vi "Lidar Processing.vi"(7 "robotPosition":T2, 8 "Direction 2":dbl[](array[numeric]), 9 "Magnitude 2":dbl[](array[numeric]), 10 "Direction":dbl[](array[numeric]), 11 "Magnitude":dbl[](array[numeric])) -> (0 "closeLidar":cluster{dbl, dbl}[](array[cluster]), 3 "Lidar Data":cluster{dbl[], dbl[]}[](graph), 4 "plotPoints":cluster{dbl, dbl}[](array[cluster]), 5 "Error":T1)   [LabVIEW 2015]
panel:
  out "Local Lidar":cluster{dbl[], dbl[]}(graph)
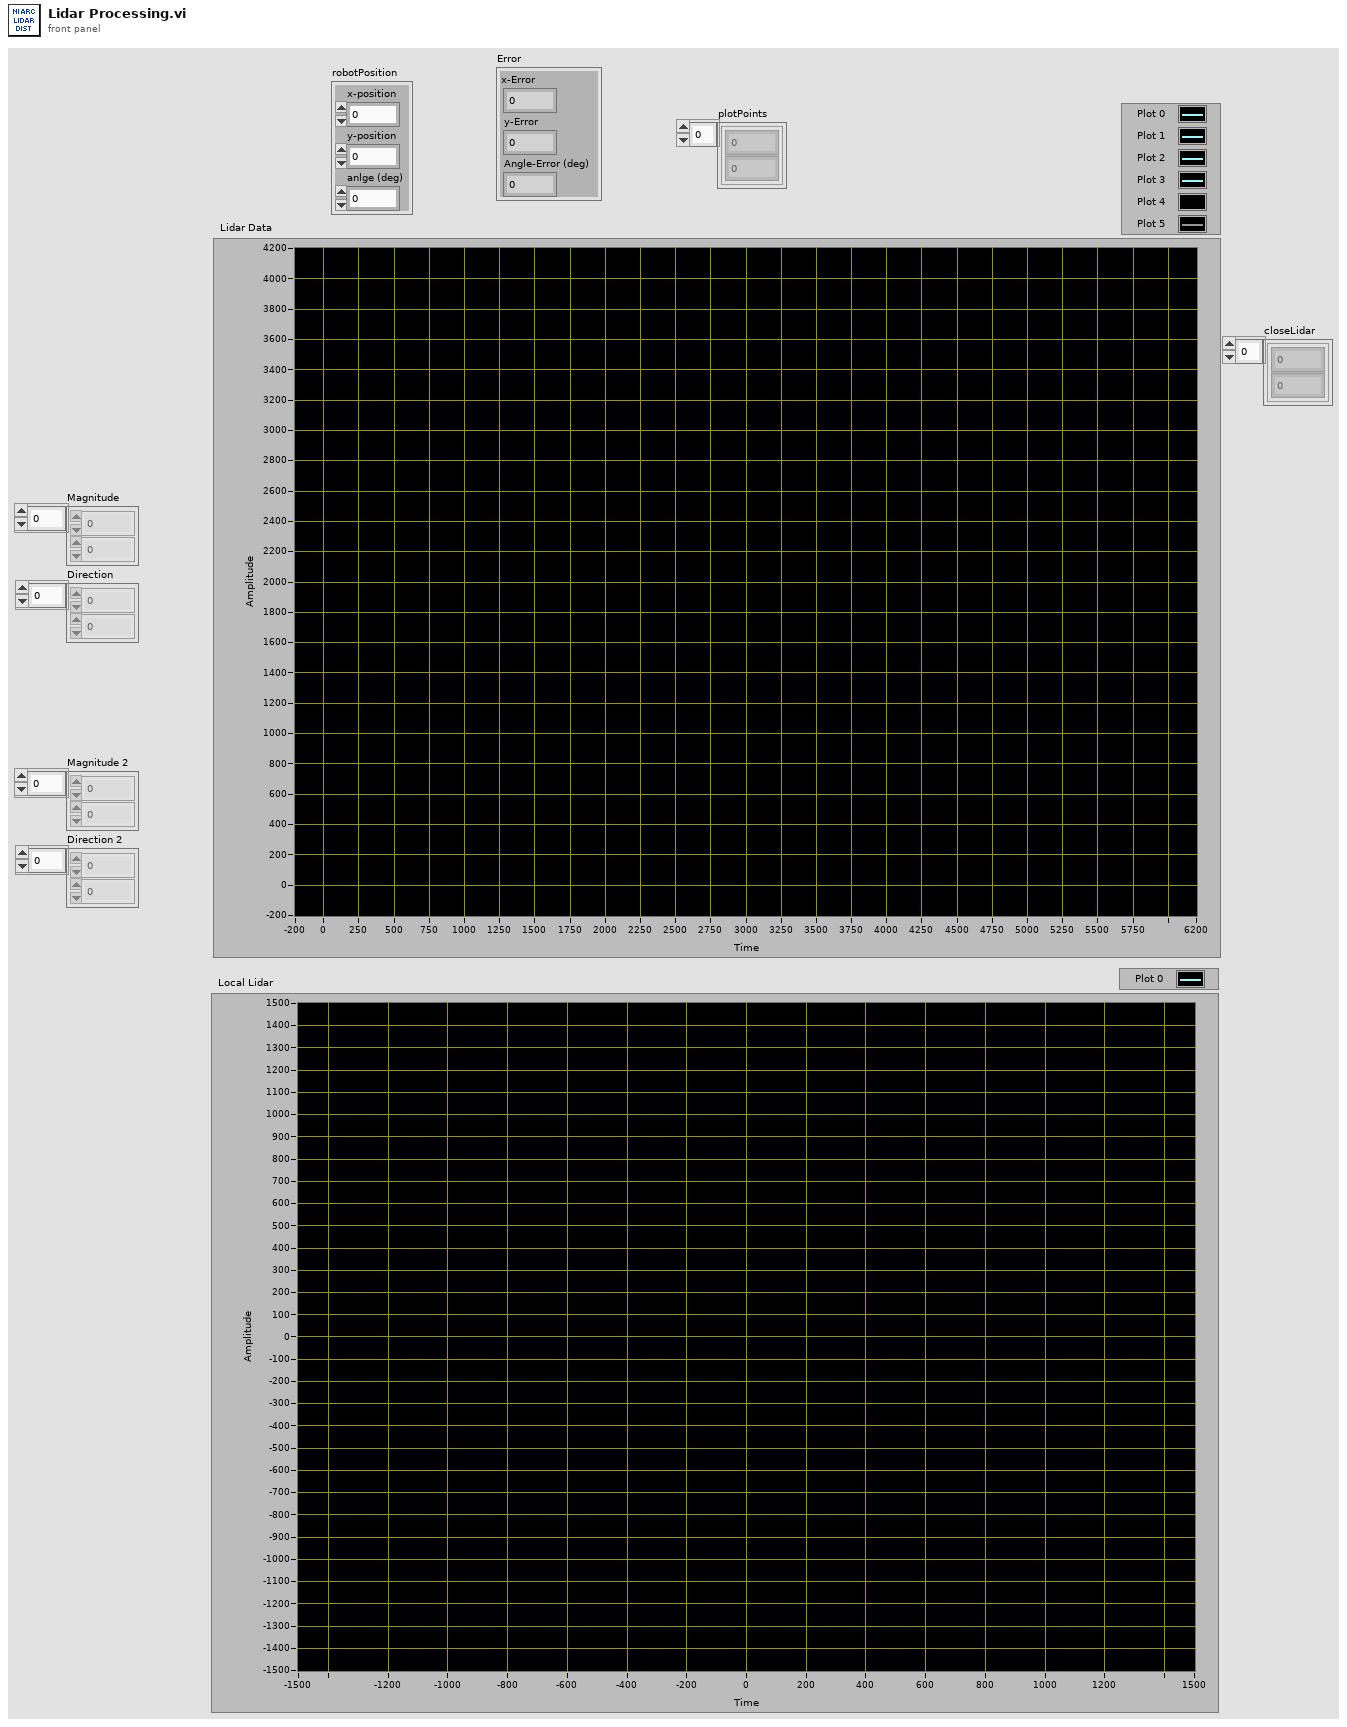
[diagram p1: front panel]
types:
  T1 = cluster{"x-Error":dbl, "y-Error":dbl, "Angle-Error (deg)":dbl}
  T2 = cluster{"x-position":dbl, "y-position":dbl, "anlge (deg)":dbl}
  T3 = cluster{"Line Segment":cluster{"Point 1":cluster{"X":sgl, "Y":sgl}, "Point 2":cluster{"X":sgl, "Y":sgl}}, "Residual":dbl, "Valid Fit?":bool}[]
  T4 = cluster{"t":dbl, "t":dbl, "detectedAngle (deg)":dbl}
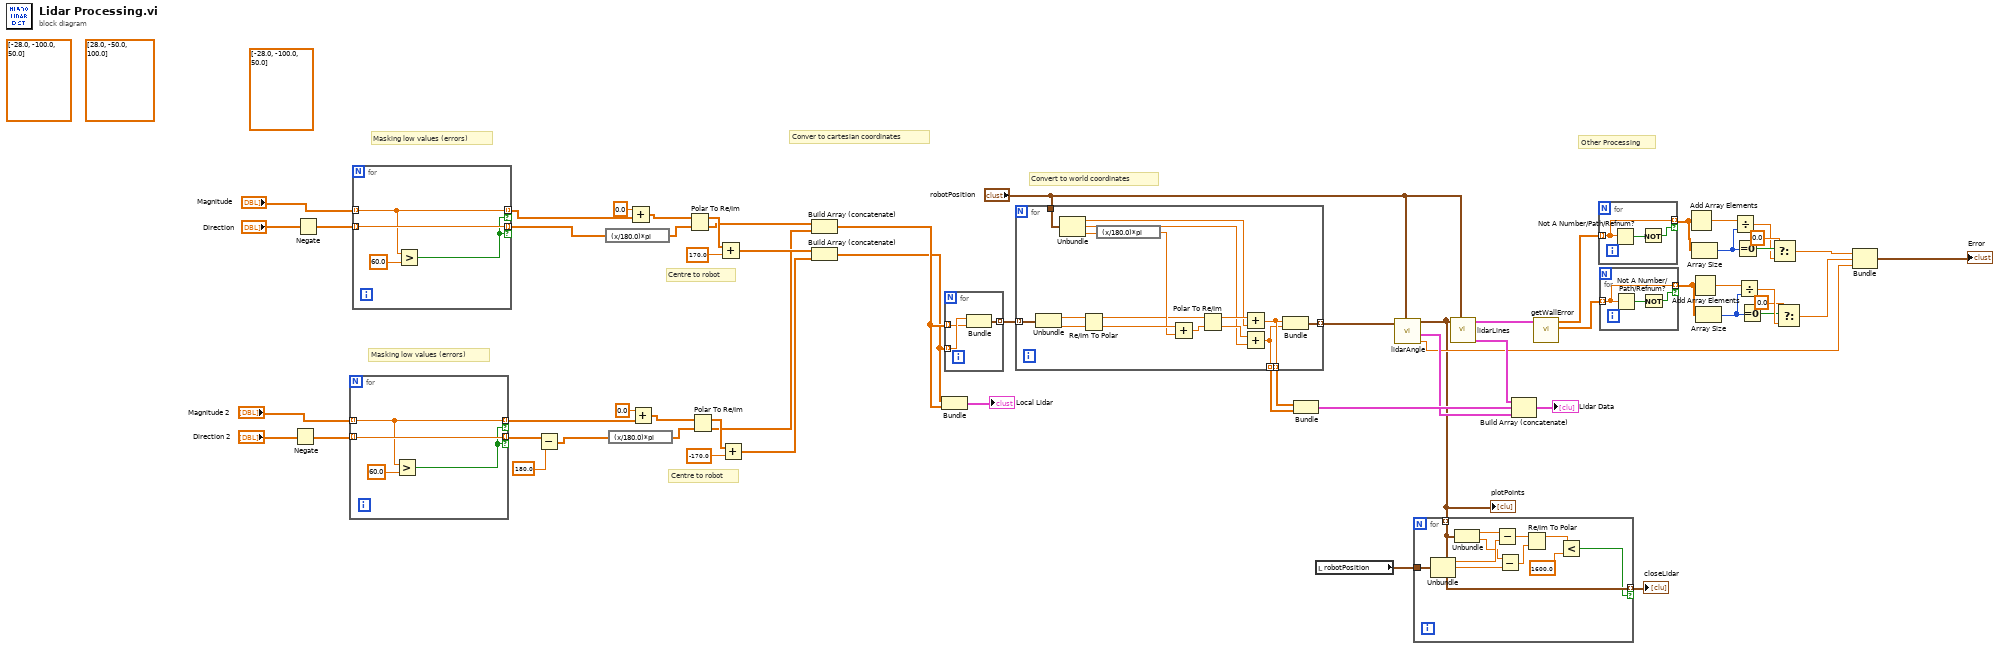
[diagram p0: block diagram]
diagram:
  (unwired) sgl[] [-28.0, -100.0, 50.0] ("Array")
  (unwired) sgl[] [28.0, -50.0, 100.0] ("Array 2")
  (unwired) sgl[] [-28.0, -100.0, 50.0] ("Array")
  # "Centre to robot"
  # "Masking low values (errors)"
  # "Convert to world coordinates"
  # "Other Processing"
  # "Masking low values (errors)"
  # "Conver to cartesian coordinates"
  # "Centre to robot"
  n1 = Negate(x="Direction 2") -> (-x=w21:dbl[])
  n2 = Negate(x="Direction") -> (-x=w56:dbl[])
  n3 = for {
    tunnel: "Magnitude 2" -> [w62] mode=indexing
    tunnel: w21 -> [w64] mode=indexing
    tunnel: [w62] -> w13 mode=indexing if=w61
    tunnel: [w64] -> w12 mode=indexing if=w61
    n4 = Greater?(x=w62, y=60.0) -> (0:w61:bool)
  }
  n5 = for {
    tunnel: "Magnitude" -> [w66] mode=indexing
    tunnel: w56 -> [w68] mode=indexing
    tunnel: [w66] -> w55 mode=indexing if=w65
    tunnel: [w68] -> w54 mode=indexing if=w65
    n6 = Greater?(x=w66, y=60.0) -> (0:w65:bool)
  }
  n7 = Subtract(x=w12, y=180.0) -> (x-y=w10:dbl[])
  n8 = expression code="(x/180.0)*pi" ("degrees to radians")(w54) -> (w59:dbl[])
  n9 = expression code="(x/180.0)*pi" ("degrees to radians")(w10) -> (w15:dbl[])
  n10 = Add(x=0.0 ("y"), y=w55) -> (x+y=w42:dbl[])
  n11 = Add(x=0.0 ("y"), y=w13) -> (x+y=w17:dbl[])
  n12 = Polar To Re/Im(2:w59, 3:w42) -> (0:w7:dbl[], 1:w53:dbl[])
  n13 = Polar To Re/Im(2:w15, 3:w17) -> (0:w4:dbl[], 1:w16:dbl[])
  n14 = Add(x=w53, y=sgl 170.0 ("n")) -> (x+y=w9:dbl[])
  n15 = Add(x=w16, y=sgl -170.0 ("n")) -> (x+y=w8:dbl[])
  n16 = Build Array (concatenate)(w7, w4) -> (w6:dbl[])
  n17 = Build Array (concatenate)(w9, w8) -> (w5:dbl[])
  n18 = Bundle(w5, w6) -> (→"Local Lidar":cluster{dbl[], dbl[]})  [unwired: 1 in]
  n19 = for {
    tunnel: w5 -> [w70] mode=indexing
    tunnel: [w71] -> w47 mode=indexing
    tunnel: w6 -> [w69] mode=indexing
    n20 = Bundle(w70, w69) -> (w71:cluster{dbl, dbl})  [unwired: 1 in]
  }
  n21 = for {
    tunnel: w47 -> [w87] mode=indexing
    tunnel: "robotPosition" -> [w86]
    tunnel: [w73] -> w46 mode=indexing
    tunnel: [w75] -> w45 mode=indexing
    tunnel: [w74] -> w44 mode=indexing
    n22 = Unbundle(w87) -> (w84:dbl, w83:dbl)
    n23 = Unbundle(w86) -> ("x-position"=w77:dbl, "y-position"=w76:dbl, "anlge (deg)"=w85:dbl)
    n24 = Re/Im To Polar(2:w83, 3:w84) -> (0:w82:dbl, 1:w72:dbl)
    n25 = expression code="(x/180.0)*pi" ("degrees to radians")(w85) -> (w81:dbl)
    n26 = Add(x=w82, y=w81) -> (x+y=w80:dbl)
    n27 = Polar To Re/Im(2:w80, 3:w72) -> (0:w78:dbl, 1:w79:dbl)
    n28 = Add(x=w79, y=w77) -> (x+y=w75:dbl)
    n29 = Add(x=w78, y=w76) -> (x+y=w74:dbl)
    n30 = Bundle(w75, w74) -> (w73:cluster{dbl, dbl})  [unwired: 1 in]
  }
  n31 = Bundle(w45, w44) -> (w52:cluster{dbl[], dbl[]})  [unwired: 1 in]
  n32 = local read "robotPosition"() -> (w2:T2)
  n33 = call "lidarAngle.vi"("robotPosition"="robotPosition", "points"=w46) -> ("detectedAngle (deg)"=w23:dbl, "plot"=w51:cluster{dbl[], dbl[]}, "correctedPoints"=w3:cluster{dbl, dbl}[])  [unwired: 7 in]
  "plotPoints" <- w3
  n34 = for {
    tunnel: w3 -> [w89] mode=indexing
    tunnel: w2 -> [w98]
    tunnel: [w89] -> w1 mode=indexing if=w88
    n35 = Unbundle(w98) -> ("x-position"=w96:dbl, "y-position"=w95:dbl)  [unwired: 1 out]
    n36 = Unbundle(w89) -> (w97:dbl, w94:dbl)
    n37 = Subtract(x=w97, y=w96) -> (x-y=w93:dbl)
    n38 = Subtract(x=w94, y=w95) -> (x-y=w92:dbl)
    n39 = Re/Im To Polar(2:w92, 3:w93) -> (1:w91:dbl)  [unwired: 1 out]
    n40 = Less?(x=w91, y=1600.0) -> (x < y?=w88:bool)
  }
  "closeLidar" <- w1
  n41 = call "lidarLines.vi"("robotPosition"="robotPosition", "points"=w3) -> ("plots"=w49:cluster{sgl[], sgl[]}[], "segments"=w48:T3)  [unwired: 8 in]
  n42 = Build Array (concatenate)(w49, w52, w51) -> (→"Lidar Data":cluster{dbl[], dbl[]}[])
  n43 = call "getWallError.vi"("segments"=w48) -> ("verticalErros"=w39:dbl[], "horizontalErrors"=w40:dbl[])  [unwired: 9 in]
  n44 = for {
    tunnel: w40 -> [w101] mode=indexing
    tunnel: [w101] -> w38 mode=indexing if=w99
    n45 = Not A Number/Path/Refnum?(number/path/refnum=w101) -> (NaN/Path/Refnum?=w100:bool)
    n46 = Not(x=w100) -> (.not. x?=w99:bool)
  }
  n47 = for {
    tunnel: w39 -> [w104] mode=indexing
    tunnel: [w104] -> w27 mode=indexing if=w102
    n48 = Not A Number/Path/Refnum?(number/path/refnum=w104) -> (NaN/Path/Refnum?=w103:bool)
    n49 = Not(x=w103) -> (.not. x?=w102:bool)
  }
  n50 = Add Array Elements(numeric array=w38) -> (sum=w37:dbl)
  n51 = Array Size(array=w38) -> (size(s)=w36:i32)
  n52 = Add Array Elements(numeric array=w27) -> (sum=w28:dbl)
  n53 = Array Size(array=w27) -> (size(s)=w29:i32)
  n54 = Divide(x=w37, y=w36) -> (x/y=w33:dbl)
  n55 = Equal To 0?(x=w36) -> (x = 0?=w35:bool)
  n56 = Divide(x=w28, y=w29) -> (x/y=w32:dbl)
  n57 = Equal To 0?(x=w29) -> (x = 0?=w30:bool)
  n58 = Select(t=0.0, s=w35, f=w33) -> (s? t:f=w26:dbl)
  n59 = Select(t=0.0, s=w30, f=w32) -> (s? t:f=w25:dbl)
  n60 = Bundle("t"=w26, "t"=w25, "detectedAngle (deg)"=w23) -> (→"Error":T4)  [unwired: 1 in]
